vi "TeslaSenseGUI Final.vi"() -> ()   [LabVIEW 2019]
uses:
  Control 5.ctl
  Global 2.vi
panel:
  in  "Clear":string[][](table)
  out "time stamp":timestamp
  in  "Server Closed":T1="The server VI closed the connection."
  in  "Connect to Server?":bool
  in  "Vibration Z":dbl=2.0
  in  "Vibration Y":dbl=2.0
  in  "Vibration X":dbl=2.0
  in  "Current":dbl=4.0
  out "Vibration":waveform(dbl)[](graph)
  out "Hall Effect Alarm":bool
  out "Vibration Alarm":bool
  out "Critical Alarm":bool
  out "No GIC Detected":bool
  out "Current  2":waveform(dbl)(graph)
  out "?":bool
  out "?":bool
  in  "Table":string[][](table)
  in  "Generate Graphs":bool
  # "TeslaSense"
  # "Threshold Configuration"
  # "GIC Data Acquisition System"
  # "Connect To Server"
  # "NO GIC DETECTED"
  # "Hall-Effect Sensor"
  # "Vibration Sensor"
  # "Critcal GIC Detected"
  # "Battery Low"
  # "SD Card Detected"
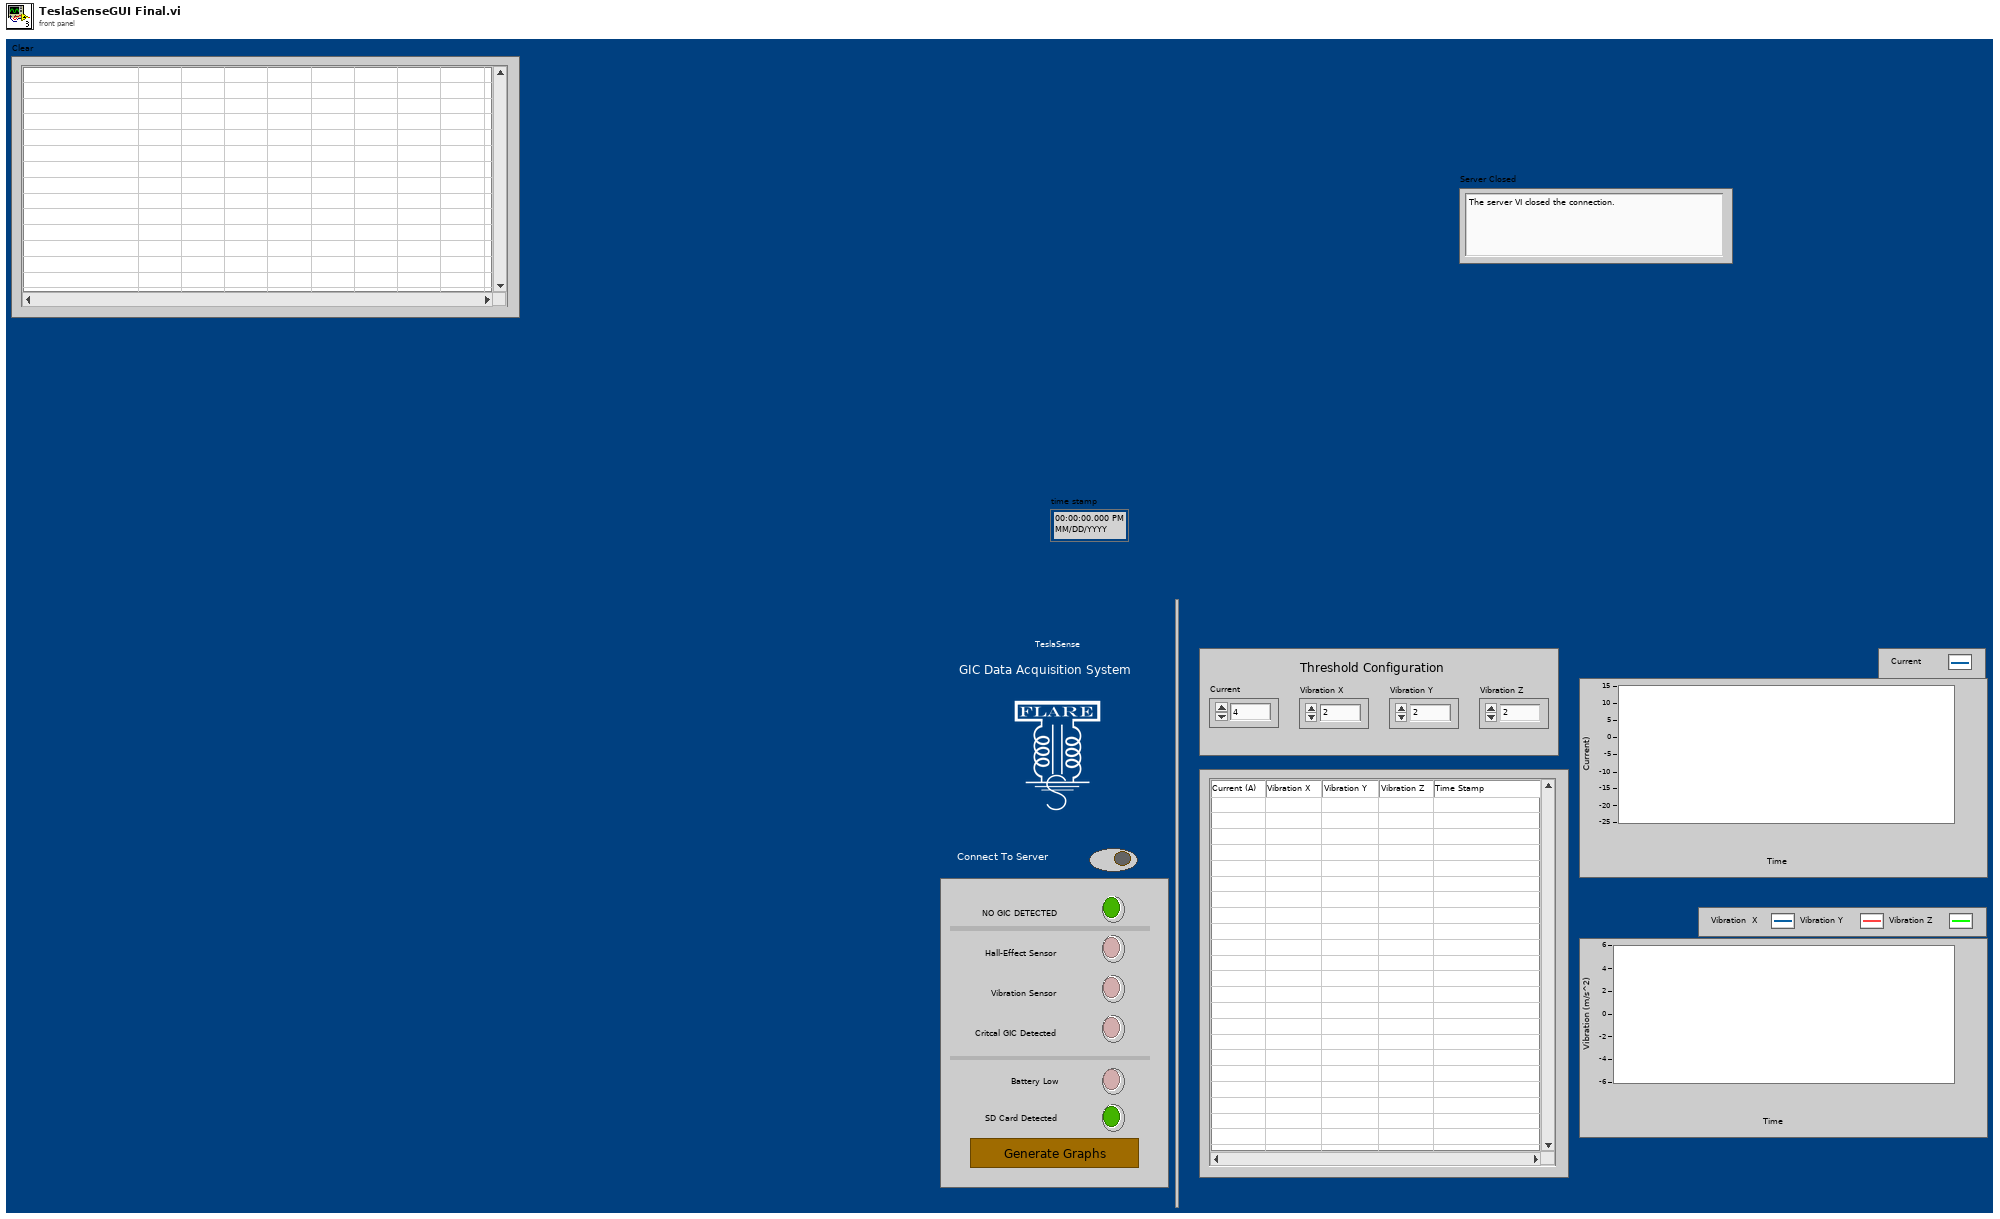
[diagram p1: front panel]
types:
  T1 = typedef "Control 5.ctl" = string
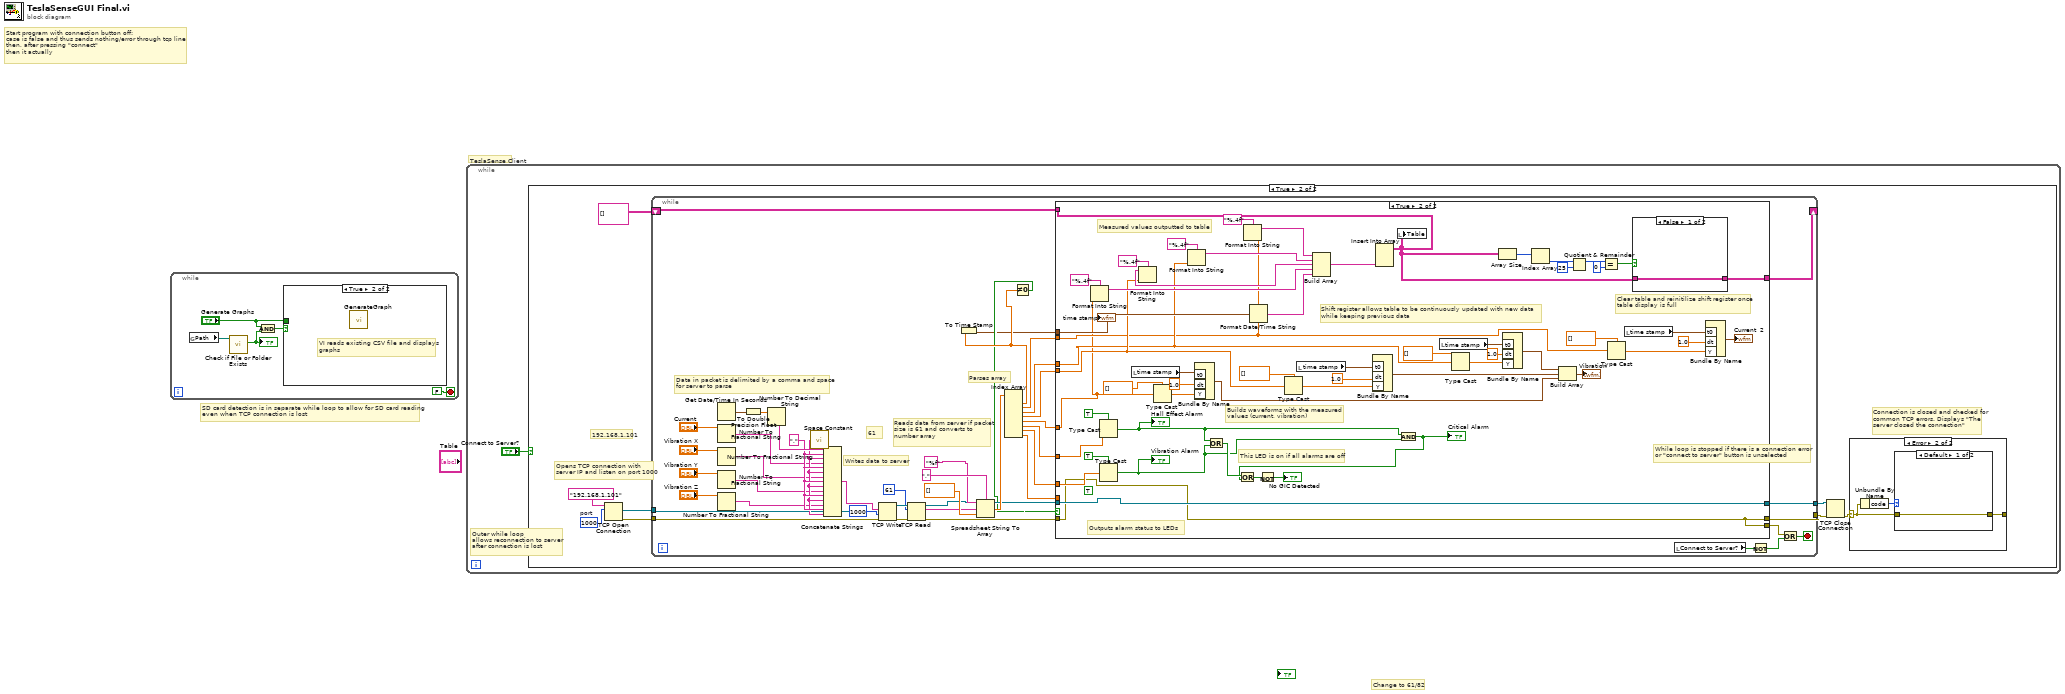
[diagram p0: block diagram]
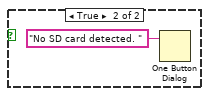
[diagram p3: hidden frame]
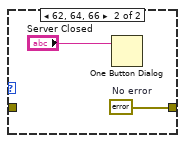
[diagram p6: hidden frame]
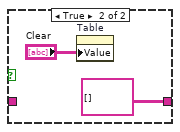
[diagram p8: hidden frame]
diagram:
  # "TeslaSense Client"
  # "SD card detection is in separate while loop to allow for SD card reading \neven when TCP connection is lost"
  # "Change to 61/82"
  # "Start program with connection button off:\ncase is false and thus sends nothing/error through tcp line \nthen, after pressing \"connect\"\nthen it actually"
  n1 = while {
    stop <- FALSE stop-if-true
    n2 = global read "Global 2.vi" "Path"() -> (w3:path)
    n3 = call <vilib>:"Check if File or Folder Exists.vi"("path"=w3) -> ("file or folder exists?"=w1:bool)  [unwired: 8 in, 2 out]
    "?" <- w1
    n4 = And(x="Generate Graphs", y=w1) -> (x .and. y?=w5:bool)
    n5 = case shown="True" w5 {
      tunnel: "Generate Graphs" -> [w6 _]
      frame False {
        # "If the file does not exist, this indicates that SD \ncard has not been inserted"
        n6 = case shown="False" w6 {
          frame False {
          }
          frame True {
            n7 = One Button Dialog(message="No SD card detected. ") -> ()  [unwired: 1 in, 1 out]
          }
        }
      }
      frame True {
        # "VI reads existing CSV file and displays \ngraphs"
        n8 = call "GenerateGraph.vi"() -> ()  [unwired: 12 in]
      }
    }
  }
  n9 = while {
    stop <- FALSE stop-if-true
    # "Outer while loop\nallows reconnection to server\nafter connection is lost"
    n10 = case shown="True" "Connect to Server?" {
      frame False {
        # "If 'Connect to server' button is not pressed, TCP handshake does not occur"
      }
      frame True {
        w16 = u16 1000  # port
        # "192.168.1.101"
        # "Connection is closed and checked for common TCP errors. Displays \"The server closed the connection\""
        # "While loop is stopped if there is a connection error \nor \"connect to server\" button is unselected"
        # "Opens TCP connection with \nserver IP and listen on port 1000"
        n11 = TCP Open Connection(address="192.168.1.101", remote port or service name=w16) -> (connection ID=w13:refnum<k5>, error out=w14:errorcluster)  [unwired: 3 in]
        n12 = while {
          shift-right: [w55] -> _
          shift-left: string[][] [] -> [w47]
          tunnel: [w53] -> w10
          tunnel: [w54] -> w11
          tunnel: w14 -> [w52]
          tunnel: w13 -> [w51]
          stop <- w46 stop-if-true
          w66 = ","
          # "Parses array"
          # "Reads data from server if packet size is 61 and converts to number array"
          # "61"
          # "Writes data to server"
          # "Data in packet is delimited by a comma and space\nfor server to parse"
          n13 = Get Date/Time In Seconds() -> (seconds since 1Jan1904=w69:timestamp)
          n14 = Number To Fractional String(number="Current") -> (F-format string=w64:string)  [unwired: 3 in]
          n15 = Number To Fractional String(number="Vibration X") -> (F-format string=w62:string)  [unwired: 3 in]
          n16 = Number To Fractional String(number="Vibration Y") -> (F-format string=w60:string)  [unwired: 3 in]
          n17 = Number To Fractional String(number="Vibration Z") -> (F-format string=w58:string)  [unwired: 3 in]
          n18 = To Double Precision Float(number=w69) -> (double precision float=w68:dbl)
          n19 = Number To Decimal String(number=w68) -> (decimal integer string=w67:string)  [unwired: 1 in]
          n20 = call <vilib>:"Space Constant.vi"() -> ("String"=w65:string)
          n21 = Concatenate Strings(w67, w66, w65, w64, w66, w65, w62, w66, w65, w60, w66, w65, w58, w66, w65) -> (w56:string)
          n22 = TCP Write(connection ID=w51, data in=w56, error in (no error)=w52, 9:1000 ("timeout ms (25000)")) -> (connection ID out=w41:refnum<k5>, error out=w39:errorcluster)  [unwired: 1 out]
          n23 = TCP Read(connection ID=w41, bytes to read=61, error in (no error)=w39) -> (connection ID out=w35:refnum<k5>, data out=w42:string, error out=w38:errorcluster)  [unwired: 2 in]
          n24 = Spreadsheet String To Array(delimiter (Tab)=",", format string="%f", spreadsheet string=w42, array type (2D Dbl)=dbl[] []) -> (array=w36:dbl[])
          n25 = Index Array(array=w36) -> (element #1=w31:dbl, element #2=w30:dbl, element #3=w29:dbl, element #4=w25:dbl, element #5=w28:dbl, element #6=w32:dbl, element #7=w33:dbl, element #8=w34:dbl)  [unwired: 8 in]
          n26 = To Time Stamp(1:w31) -> (0:w26:timestamp)
          n27 = Not Equal To 0?(x=w31) -> (x != 0?=w27:bool)
          n28 = case shown="True" w27 {
            tunnel: [w72 w78] -> w54
            tunnel: w35 -> [w72 w78]
            tunnel: w38 -> [w70 w76]
            tunnel: [w70 w76] -> w53
            tunnel: w47 -> [w71 w110]
            tunnel: [w71 w86] -> w55
            tunnel: [w70 w76] -> w49
            tunnel: w26 -> [_ w84]
            tunnel: w34 -> [_ _]
            tunnel: w33 -> [_ w83]
            tunnel: w32 -> [_ w82]
            tunnel: w30 -> [_ w79]
            tunnel: w29 -> [_ w80]
            tunnel: w25 -> [_ w81]
            tunnel: w28 -> [_ w77]
            frame False {
              # "The server has not written any data"
            }
            frame True {
              (unwired) TRUE
              # "Clear table and reinitilize shift register once table display is full"
              # "Measured values outputted to table"
              # "Builds waveforms with the measured values (current, vibration)"
              # "Outputs alarm status to LEDs"
              # "Shift register allows table to be continuously updated with new data\nwhile keeping previous data"
              # "This LED is on if all alarms are off"
              n29 = Format Into String(format string="%.4f", w77) -> (resulting string=w97:string)  [unwired: 2 in, 1 out]
              n30 = Type Cast(type=TRUE, x=w82) -> (*(type *) &x=w75:bool)
              "Hall Effect Alarm" <- w75
              n31 = Type Cast(type=TRUE, x=w83) -> (*(type *) &x=w74:bool)
              "Vibration Alarm" <- w74
              n32 = local read "time stamp"() -> (w107:timestamp)
              n33 = Format Into String(format string="%.4f", w81) -> (resulting string=w98:string)  [unwired: 2 in, 1 out]
              n34 = Type Cast(type=dbl[] [], x=w77) -> (*(type *) &x=w119:dbl[])
              n35 = Format Into String(format string="%.4f", w80) -> (resulting string=w99:string)  [unwired: 2 in, 1 out]
              n36 = Bundle By Name("t0"=w107, "dt"=1.0, "Y"=w119) -> (w94:waveform(dbl))  [unwired: 1 in]
              n37 = Or(x=w75, y=w74) -> (x .or. y?=w116:bool)
              n38 = Format Into String(format string="%.4f", w79) -> (resulting string=w95:string)  [unwired: 2 in, 1 out]
              n39 = Format Date/Time String(seconds (now)=w84) -> (date/time string=w113:string)  [unwired: 2 in]
              n40 = Type Cast(type=dbl[] [], x=w81) -> (*(type *) &x=w105:dbl[])
              n41 = local read "time stamp"() -> (w106:timestamp)
              n42 = Build Array(w95, w99, w98, w97, w113) -> (w112:string[])
              n43 = Bundle By Name("t0"=w106, "dt"=1.0, "Y"=w105) -> (w121:waveform(dbl))  [unwired: 1 in]
              n44 = Insert Into Array(array=w110, new element=w112) -> (w87:string[][])  [unwired: 2 in]
              n45 = local write "Table"(w87) -> ()
              n46 = And(x=w75, y=w74) -> (x .and. y?=w73:bool)
              "Critical Alarm" <- w73
              n47 = Or(x=w116, y=w73) -> (x .or. y?=w115:bool)
              n48 = Not(x=w115) -> (.not. x?=→"No GIC Detected":bool)
              n49 = local read "time stamp"() -> (w104:timestamp)
              n50 = Type Cast(type=dbl[] [], x=w80) -> (*(type *) &x=w125:dbl[])
              n51 = Array Size(array=w87) -> (size(s)=w93:i32[])
              n52 = Bundle By Name("t0"=w104, "dt"=1.0, "Y"=w125) -> (w124:waveform(dbl))  [unwired: 1 in]
              n53 = Index Array(array=w93) -> (element=w91:i32)  [unwired: 1 in]
              n54 = Build Array(w124, w121, w94) -> (→"Vibration":waveform(dbl)[])
              n55 = Quotient & Remainder(x=w91, y=25) -> (x-y*floor(x/y)=w89:i32)  [unwired: 1 out]
              n56 = Equal?(x=w89, y=0) -> (x = y?=w92:bool)
              n57 = Type Cast(type=dbl[] [], x=w79) -> (*(type *) &x=w128:dbl[])
              n58 = local read "time stamp"() -> (w108:timestamp)
              n59 = case shown="False" w92 {
                tunnel: [w130 string[][] []] -> w86
                tunnel: w87 -> [w130 _]
                frame False {
                }
                frame True {
                  n60 = property on="Table" class="Tbl (strict)"("Value"="Clear") -> ()  [unwired: 2 in, 2 out]
                }
              }
              n61 = Bundle By Name("t0"=w108, "dt"=1.0, "Y"=w128) -> (→"Current  2":waveform(dbl))  [unwired: 1 in]
              "time stamp" <- w84
            }
          }
          n62 = local read "Connect to Server?"() -> (w50:bool)
          n63 = Not(x=w50) -> (.not. x?=w48:bool)
          n64 = Or(x=w49, y=w48) -> (x .or. y?=w46:bool)
        }
        n65 = TCP Close Connection(connection ID=w11, error in (no error)=w10) -> (error out=w12:errorcluster)  [unwired: 1 in, 1 out]
        n66 = case shown="Error" w12 {
          selector: w12 -> [w18 w20]
          tunnel: [w18 w19] -> _
          frame No Error {
          }
          frame Error {
            n67 = Unbundle By Name(w20) -> ("code"=w21:i32)
            n68 = case shown="Default" w21 {
              tunnel: w20 -> [w22 _]
              tunnel: [w22 w24] -> w19
              frame Default {
              }
              frame 62, 64, 66 {
                w24 = errorcluster {"status"=FALSE, "code"=0, "source"=""}  # No error
                n69 = One Button Dialog(message="Server Closed") -> ()  [unwired: 1 in, 1 out]
              }
            }
          }
        }
      }
    }
  }
